vi "Wfm przesun ramki do linii.vi"(6 "Plot Bounds":T1[](array[typedef]), 8 "error in (no error)":errorcluster, 11 "Wfm Refs in":refnum<vi>[](array[refnum])) -> (0 "error out":errorcluster, 3 "Wfm Refs out":refnum<vi>[](array[refnum]))   [LabVIEW 2014]
uses:
  <vilib>/Utility/miscctls.llb/LVRectTypeDef.ctl
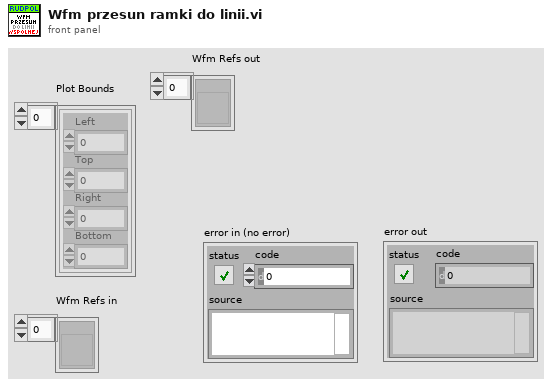
[diagram p1: front panel]
types:
  T1 = typedef "LVRectTypeDef.ctl" = cluster{"Left":i16, "Top":i16, "Right":i16, "Bottom":i16}
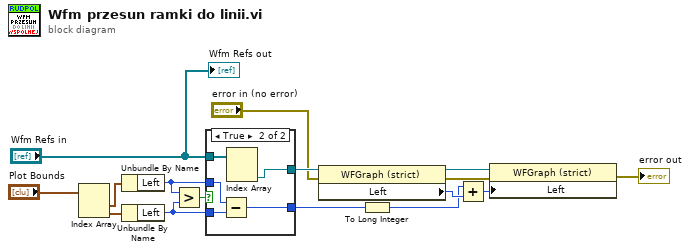
[diagram p0: block diagram]
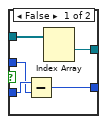
[diagram p2: hidden frame]
diagram:
  n1 = Index Array(array="Plot Bounds") -> (element #1=w11:T1, element #2=w12:T1)  [unwired: 2 in]
  n2 = Unbundle By Name(w11) -> ("Left"=w14:i16)
  n3 = Unbundle By Name(w12) -> ("Left"=w15:i16)
  n4 = Greater?(x=w14, y=w15) -> (0:w13:bool)
  n5 = case shown="True" w13 {
    tunnel: w14 -> [w20 w25]
    tunnel: w15 -> [w21 w26]
    tunnel: "Wfm Refs in" -> [w19 w24]
    tunnel: [w18 w23] -> w7
    tunnel: [w17 w22] -> w3
    frame False {
      n6 = Subtract(x=w21, y=w20) -> (x-y=w17:i16)
      n7 = Index Array(array=w19) -> (element #1=w18:refnum<vi>)  [unwired: 2 in, 1 out]
    }
    frame True {
      n8 = Subtract(x=w25, y=w26) -> (x-y=w22:i16)
      n9 = Index Array(array=w24) -> (element #2=w23:refnum<vi>)  [unwired: 2 in, 1 out]
    }
  }
  n10 = property class="WFGraph (strict)"(reference=w7, error in="error in (no error)") -> (reference out=w9:refnum<vi>, error out=w6:errorcluster, "Left"=w8:i32)
  n11 = To Long Integer(number=w3) -> (32bit integer=w2:i32)
  n12 = Add(x=w2, y=w8) -> (x+y=w10:i32)
  n13 = property class="WFGraph (strict)"(reference=w9, error in=w6, "Left"=w10) -> (error out=→"error out":errorcluster)  [unwired: 1 out]
  "Wfm Refs out" <- "Wfm Refs in"
